vi "Index Array (Object).vi"(8 "error in (no error)":errorcluster, 9 "index":i32, 10 "JSON Array in":refnum<class "JSON Array.lvclass">) -> (0 "error out":errorcluster, 1 "JSON Object":refnum<class "JSON Object.lvclass">)   [LabVIEW 2015, in "LVJSON.lvlib" / "JSON Array.lvclass"]
uses:
  JSON Array.lvclass
  JSON Object/JSON Object.lvclass
  JSON Helper/To More Specific Type (Object).vi
  JSON Helper/JSON Helper.lvclass
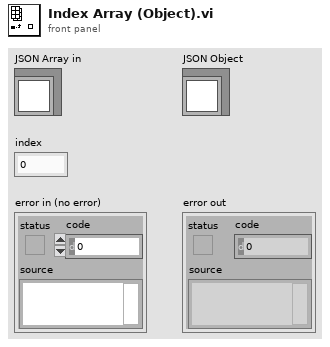
[diagram p1: front panel]
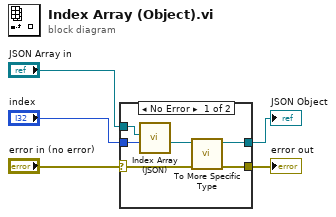
[diagram p0: block diagram]
diagram:
  n1 = case shown="No Error" "error in (no error)" {
    selector: "error in (no error)" -> [w9 w12]
    tunnel: [w8 w12] -> w4
    tunnel: "JSON Array in" -> [w10 _]
    tunnel: "index" -> [w11 _]
    tunnel: [w6 _] -> w1
    frame No Error {
      n2 = call "Index Array (JSON).vi"("index"=w11, "JSON Array in"=w10) -> ("JSON Data"=w7:refnum<class "JSON Null.lvclass">)  [unwired: 9 in]
      n3 = call-poly "To More Specific Type.vi"("error in (no error)"=w9, "JSON Datatype in"=w7) -> ("error out"=w8:errorcluster, "JSON Datatype out"=w6:refnum<class "JSON Object.lvclass">)  [unwired: 8 in]
    }
    frame Error {
    }
  }
  "error out" <- w4
  "JSON Object" <- w1
